vi "Analog_Output_4Channels_W20I5.vi"(1 "Values":fxp<+/-,20,5>[](array[numeric])=[0.0, 0.0, 0.0, 0.0], 2 "IO":T1={"AO 0"="Connector1/AO0", "AO 1"="Connector1/AO0", "AO 2"="Connector1/AO0", "AO 3"="Connector1/AO0"}) -> ()   [LabVIEW 2015]
uses:
  <vilib>/rvi/eio/common/nirviEmuTemplateMethod_errors.vi
  <vilib>/eio/EIONode/EIONode.xnode
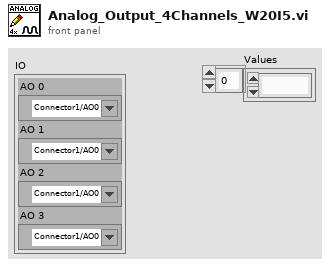
[diagram p1: front panel]
types:
  T1 = cluster{"AO 0":refnum<k21>, "AO 1":refnum<k21>, "AO 2":refnum<k21>, "AO 3":refnum<k21>}
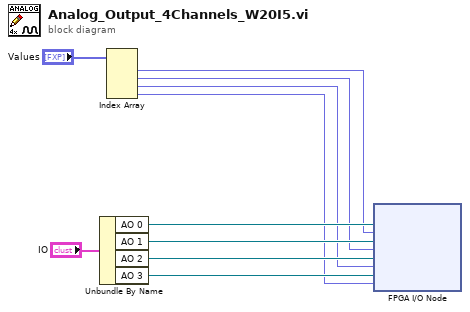
[diagram p0: block diagram]
diagram:
  n1 = Unbundle By Name("IO") -> ("AO 0"=w9:refnum<k21>, "AO 1"=w8:refnum<k21>, "AO 2"=w7:refnum<k21>, "AO 3"=w6:refnum<k21>)
  n2 = Index Array(array="Values") -> (element #1=w4:fxp<+/-,20,5>, element #2=w3:fxp<+/-,20,5>, element #3=w2:fxp<+/-,20,5>, element #4=w1:fxp<+/-,20,5>)  [unwired: 4 in]
  n3 = xnode "FPGA I/O Node"("I/O Item"=w4, "FPGA I/O In"=w9, "I/O Item"=w3, "FPGA I/O In"=w8, "I/O Item"=w2, "FPGA I/O In"=w7, "I/O Item"=w1, "FPGA I/O In"=w6) -> ()  [unwired: 4 out]
